vi "Phasics analyze.vi"(8 "error in (no error)":errorcluster, 10 "Image in":i16[][](array[numeric]), 11 "Phasics Camera in":refnum<class "Phasics Camera.lvclass">) -> (0 "error out":errorcluster, 3 "Phasics Camera out":refnum<class "Phasics Camera.lvclass">)   [LabVIEW 2013, in "Phasics Camera.lvclass"]
uses:
  Phasics Camera.lvclass
  Phasics Camera.lvclass/Phasics Camera.ctl
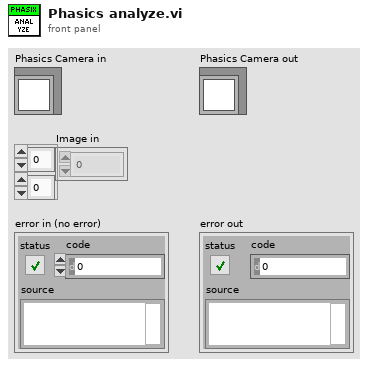
[diagram p1: front panel]
types:
  T1 = typedef "OnOffTypeDef.ctl" = enum16{"off", "on"}
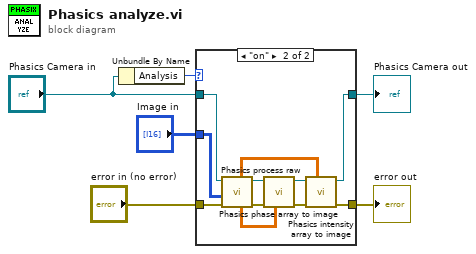
[diagram p0: block diagram]
diagram:
  n1 = Unbundle By Name("Phasics Camera in") -> ("Analysis"=w6:T1)
  n2 = case shown="\"on\"" w6 {
    tunnel: "Image in" -> [_ w19]
    tunnel: "Phasics Camera in" -> [w8 w16]
    tunnel: [w8 w15] -> w2
    tunnel: "error in (no error)" -> [w7 w13]
    tunnel: [w7 w11] -> w4
    frame "off", Default {
    }
    frame "on" {
      n3 = call "Phasics process raw.vi"("error in (no error)"=w13, "Image in"=w19, "Phasics Camera in"=w16) -> ("error out"=w12:errorcluster, "Phasics Camera out"=w14:refnum<class "Phasics Camera.lvclass">, "Phase out"=w9:sgl[][], "Intensity out"=w10:sgl[][])  [unwired: 5 in]
      n4 = call "Phasics phase array to image.vi"("Phase in"=w9, "error in (no error)"=w12, "Phasics Camera in"=w14) -> ("error out"=w18:errorcluster, "Phasics Camera out"=w17:refnum<class "Phasics Camera.lvclass">)  [unwired: 7 in]
      n5 = call "Phasics intensity array to image.vi"("Intensity in"=w10, "error in (no error)"=w18, "Phasics Camera in"=w17) -> ("error out"=w11:errorcluster, "Phasics Camera out"=w15:refnum<class "Phasics Camera.lvclass">)  [unwired: 7 in]
    }
  }
  "error out" <- w4
  "Phasics Camera out" <- w2
